vi "Collect Param - String.vi"(8 "Error in":errorcluster caption="Error in (no error)", 9 "Value":string, 10 "Param Name":string, 11 "Params Array In":T1[](array[typedef])) -> (0 "Error out":errorcluster, 3 "Params Array Out":T1[](array[typedef]))   [LabVIEW 2018]
uses:
  TypeDef/Param.ctl
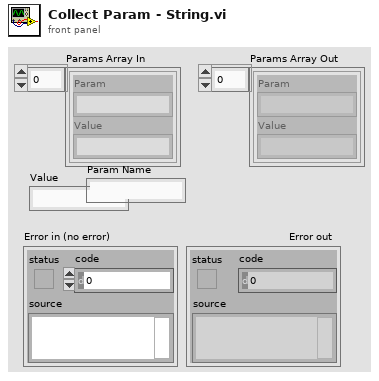
[diagram p1: front panel]
types:
  T1 = typedef "Param.ctl" = cluster{"Param":string, "Value":string}
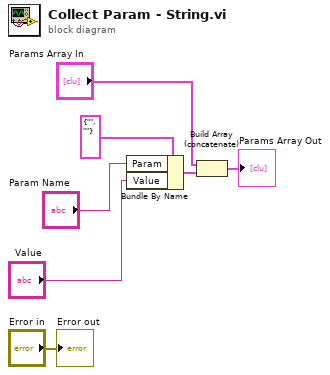
[diagram p0: block diagram]
diagram:
  n1 = Bundle By Name(cluster=T1 {"Param"="", "Value"=""} ("Cluster"), "Param"="Param Name", "Value"="Value") -> (w3:T1)
  n2 = Build Array (concatenate)("Params Array In", w3) -> (→"Params Array Out":T1[])
  "Error out" <- "Error in"
